vi "rad_Retrieve Image Wrapper.vi"(7 "Deployment Notifiers":T6, 8 "error in (no error)":errorcluster, 9 "AppImage Properties":T3, 10 "image file path":path, 11 "Target settings":T1={"Hostname"="", "Serial number"="", "Product name"="", "Product code"=0, "System status"="", "Credential type"=enum."None/Unlocked", "User added?"=FALSE, "Primary NIC"={"MAC address"="", "IP Address Request Mode"=2, "IP address"="", "Subnet mask"="", "Gateway"="", "DNS server"=""}} {"Primary NIC"."IP Address Request Mode" items=["Static"=1, "DHCP/Link-Local"=2, "Link-Local Only"=4, "DHCP Only"=8]}) -> (0 "error out":errorcluster, 3 "Canceled":bool)   [LabVIEW 2013]
uses:
  TypeDefs/rad_Deployment Progress Data Type.ctl
  TypeDefs/rad_Deployment Notifiers.ctl
  TypeDefs/rad_Deployment Status Data Type.ctl
  TypeDefs/rad_Application Image Properties.ctl
  TypeDefs/rad_FPGA Properties.ctl
  TypeDefs/rad_FPGA Flash Properties.ctl
  Targets/TypeDefs/rad_Target Information.ctl
  Targets/TypeDefs/rad_Target Network Settings.ctl
  <vilib>/nisyscfg/Software 1.2.ctl
  <vilib>/nisyscfg/Component Type.ctl
  <vilib>/nisyscfg/Create System Image (Folder).vi
  <vilib>/nisyscfg/Close (System).vi
  <vilib>/nisyscfg/nisyscfg.lvlib
panel:
  in  "Stop Checking for Events":bool
  out "Progress":T7 scale=0.0..100.0
  out "Status":string
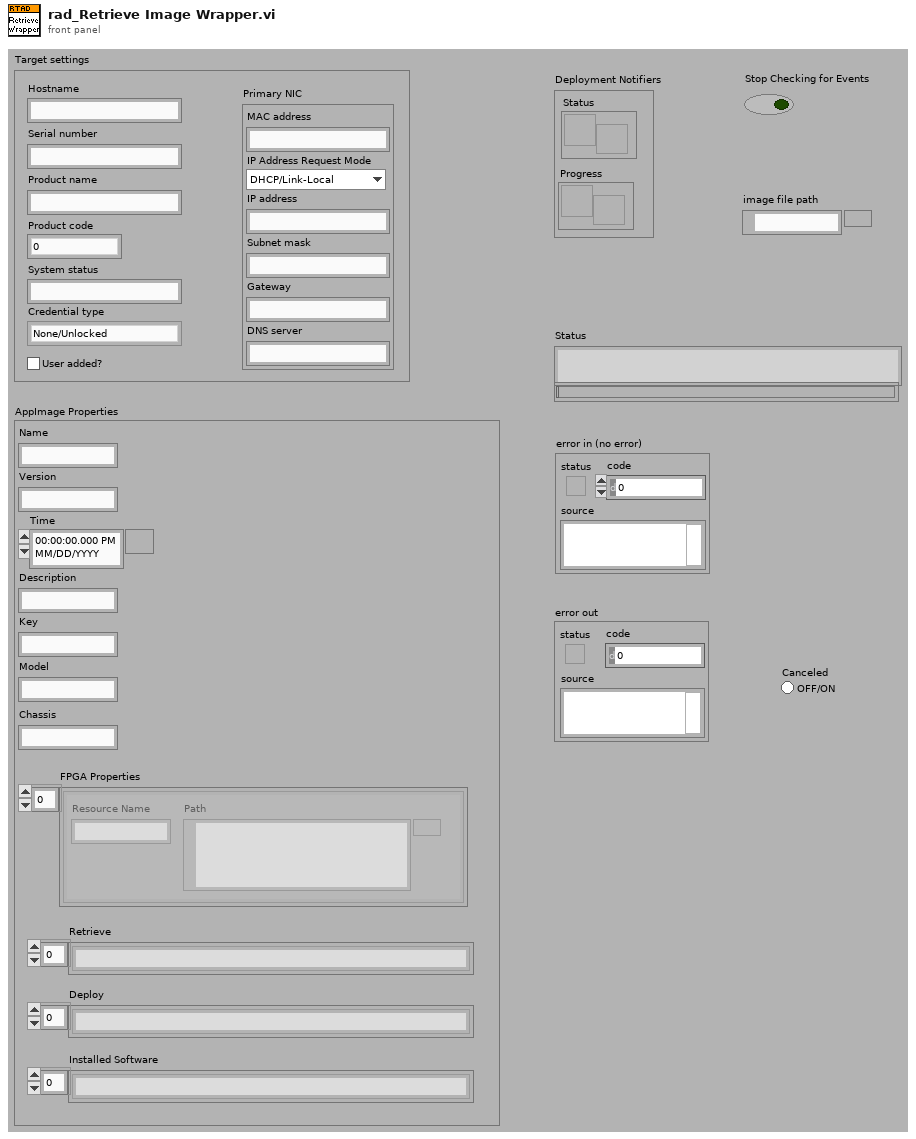
[diagram p1: front panel]
types:
  T1 = typedef "rad_Target Information.ctl" = cluster{"Hostname":string, "Serial number":string, "Product name":string, "Product code":i32, "System status":string, "Credential type":enum16{"None/Unlocked", "FTP Password", "NIAuth Credentials"}, "User added?":bool, "Primary NIC":T2}
  T2 = typedef "rad_Target Network Settings.ctl" = cluster{"MAC address":string, "IP Address Request Mode":i32, "IP address":string, "Subnet mask":string, "Gateway":string, "DNS server":string}
  T3 = typedef "rad_Application Image Properties.ctl" = cluster{"Name":string, "Version":string, "Time":timestamp, "Description":string, "Key":string, "Chassis":string, "FPGA Properties":T4, "Model":string, "Retrieve":string[], "Deploy":string[], "Installed Software":string[]}
  T4 = typedef "rad_FPGA Properties.ctl" = T5[]
  T5 = typedef "rad_FPGA Flash Properties.ctl" = cluster{"Resource Name":string, "Path":path}
  T6 = typedef "rad_Deployment Notifiers.ctl" = cluster{"Status":refnum<notifier>, "Progress":refnum<notifier>}
  T7 = typedef "rad_Deployment Progress Data Type.ctl" = i8
  T8 = typedef "nisyscfg.lvlib/Software 1.2.ctl" = cluster{"title":string, "description":string, "ID":string, "version":string, "component type":T9}
  T9 = typedef "nisyscfg.lvlib/Component Type.ctl" = u32
  T10 = enum32{"state changed", "beginning restart", "getting file", "putting file", "creating directory", "deleting file", "deleting directory", "enumerating file system", "renaming file", "current component", "operation progress", "downloading file", "unpacking file", "running install script"}
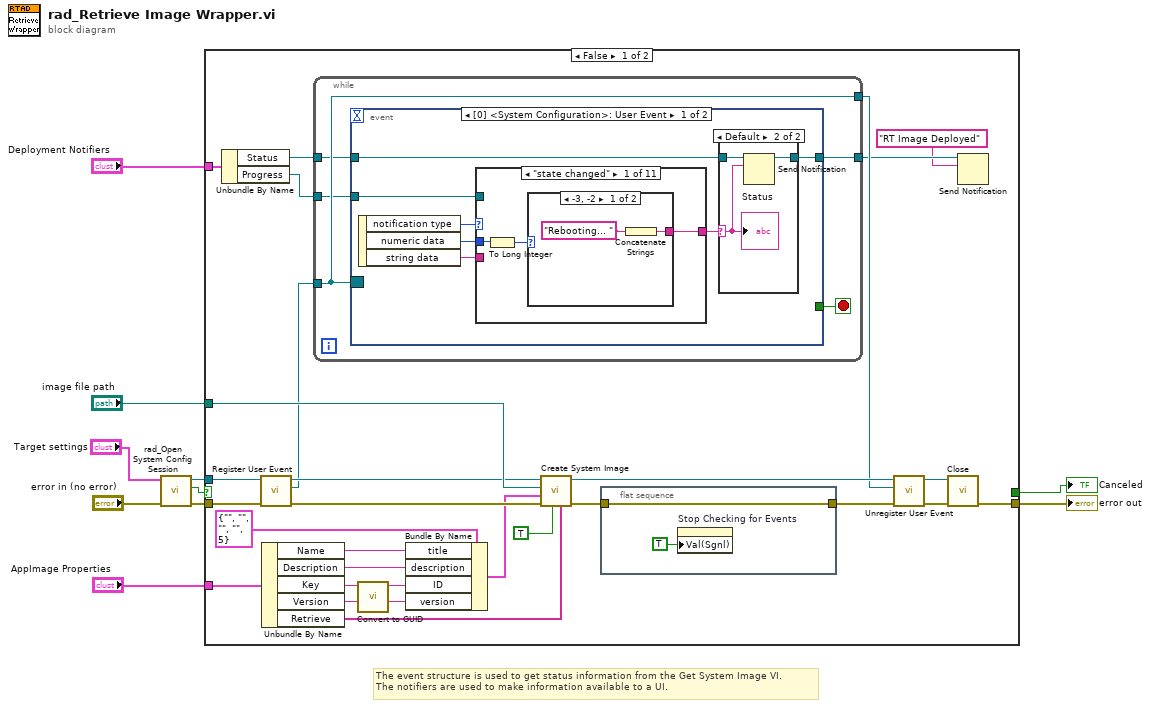
[diagram p0: block diagram]
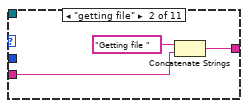
[diagram p4: hidden frame]
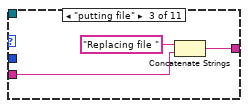
[diagram p5: hidden frame]
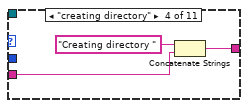
[diagram p6: hidden frame]
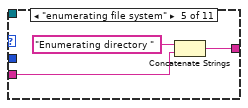
[diagram p7: hidden frame]
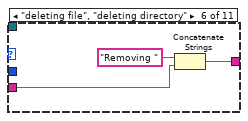
[diagram p8: hidden frame]
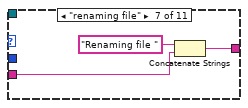
[diagram p9: hidden frame]
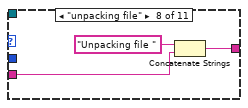
[diagram p10: hidden frame]
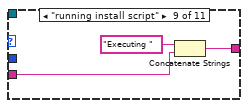
[diagram p11: hidden frame]
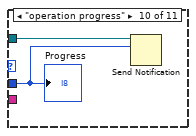
[diagram p12: hidden frame]
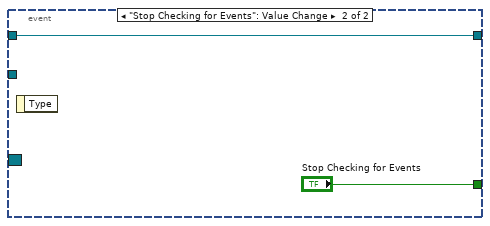
[diagram p14: hidden frame]
diagram:
  # "The event structure is used to get status information from the Get System Image VI. \nThe notifiers are used to make information available to a UI."
  n1 = call "rad_Open System Config Session.vi"("error in (no error)"="error in (no error)", "Target settings"="Target settings") -> ("error out"=w3:errorcluster, "Cancelled"=w2:bool, "Session out"=w4:refnum<k21>)  [unwired: 6 in, 1 out]
  n2 = case shown="False" w2 {
    selector: w2 -> [_ w90]
    tunnel: [w38 w91] -> w8
    tunnel: "image file path" -> [w37 _]
    tunnel: w4 -> [w36 _]
    tunnel: w3 -> [w35 w91]
    tunnel: "Deployment Notifiers" -> [w20 _]
    tunnel: "AppImage Properties" -> [w19 _]
    tunnel: [_ w90] -> w6
    frame False {
      n3 = Unbundle By Name(w20) -> ("Status"=w22:refnum<notifier>, "Progress"=w21:refnum<notifier>)
      n4 = call <vilib>:"Register User Event.vi"("error in (no error)"=w35, "Session in"=w36) -> ("error out"=w33:errorcluster, "Event Registration out"=w32:refnum<event-registration>, "Session out"=w34:refnum<k21>)  [unwired: 7 in]
      n5 = Unbundle By Name(w19) -> ("Name"=w16:string, "Description"=w15:string, "Key"=w12:string, "Version"=w14:string, "Retrieve"=w18:string[])
      n6 = while {
        tunnel: w32 -> [w45]
        tunnel: [w45] -> w28
        tunnel: w22 -> [w43]
        tunnel: [w42] -> w25
        tunnel: w21 -> [w41]
        stop <- w44 stop-if-true
        n7 = event shown="[0] <System Configuration>: User Event" {
          selector: w45 -> [_ _]
          dyn-events: _ -> [_ _]
          timeout: _ -> [_ _]
          tunnel: [_ "Stop Checking for Events"] -> w44
          tunnel: w43 -> [w48 w88]
          tunnel: [w47 w88] -> w42
          tunnel: w41 -> [w46 _]
          event User Event {
            n8 = event-data() -> ("notification type"=w52:T10, "numeric data"=w50:u32, "string data"=w51:string)  [unwired: 1 in]
            n9 = case shown="\"state changed\"" w52 {
              tunnel: [w57 w62 w65 w68 w71 w74 w77 w80 w83 _ _] -> w49
              tunnel: w51 -> [_ w63 w66 w69 w72 w75 w78 w81 w84 _ _]
              tunnel: w50 -> [w59 _ _ _ _ _ _ _ _ w86 _]
              tunnel: w46 -> [_ _ _ _ _ _ _ _ _ w87 _]
              frame "state changed" {
                n10 = To Long Integer(number=w59) -> (32bit integer=w58:i32)
                n11 = case shown="-3, -2" w58 {
                  tunnel: [w60 _] -> w57
                  frame -3, -2 {
                    n12 = Concatenate Strings("Rebooting... ") -> (w60:string)
                  }
                  frame Default {
                  }
                }
              }
              frame "getting file" {
                n13 = Concatenate Strings("Getting file " ("Status"), w63) -> (w62:string)
              }
              frame "putting file" {
                n14 = Concatenate Strings("Replacing file " ("Status"), w66) -> (w65:string)
              }
              frame "creating directory" {
                n15 = Concatenate Strings("Creating directory " ("Status"), w69) -> (w68:string)
              }
              frame "enumerating file system" {
                n16 = Concatenate Strings("Enumerating directory " ("Status"), w72) -> (w71:string)
              }
              frame "deleting file", "deleting directory" {
                n17 = Concatenate Strings("Removing " ("Status"), w75) -> (w74:string)
              }
              frame "renaming file" {
                n18 = Concatenate Strings("Renaming file " ("Status"), w78) -> (w77:string)
              }
              frame "unpacking file" {
                n19 = Concatenate Strings("Unpacking file " ("Status"), w81) -> (w80:string)
              }
              frame "running install script" {
                n20 = Concatenate Strings("Executing " ("Status"), w84) -> (w83:string)
              }
              frame "operation progress" {
                n21 = Send Notification(notification=w86, notifier=w87) -> ()  [unwired: 1 in, 2 out]
                "Progress" <- w86
              }
              frame Default {
              }
            }
            n22 = case shown="Default" w49 {
              selector: w49 -> [_ w55]
              tunnel: w48 -> [w53 w56]
              tunnel: [w53 w54] -> w47
              frame "" {
              }
              frame Default {
                n23 = Send Notification(notification=w55, notifier=w56) -> (notifier out=w54:refnum<notifier>)  [unwired: 1 in, 1 out]
                "Status" <- w55
              }
            }
          }
          event "Stop Checking for Events": Value Change {
            n24 = event-data() -> ()  [unwired: 1 in, 1 out]
          }
        }
      }
      n25 = call "Convert to GUID.vi"("Key"=w12) -> ("GUID"=w11:string)  [unwired: 10 in]
      n26 = Bundle By Name(cluster=T8 {"title"="", "description"="", "ID"="", "version"="", "component type"=5} ("image metadata"), "title"=w16, "description"=w15, "ID"=w11, "version"=w14) -> (w13:T8)
      n27 = call-poly <vilib>:"Create System Image.vi"("File and Directory Blacklist"=w18, "Overwrite (F)"=TRUE ("overwrite (F)"), "error in (no error)"=w33, "Image Metadata in"=w13, "Destination Folder"=w37, "Session in"=w34) -> ("error out"=w27:errorcluster, "Session out"=w29:refnum<k21>)  [unwired: 3 in, 1 out]
      n28 = flat-sequence {
        tunnel: w27 -> [w40]
        tunnel: [w40] -> w26
        frame #0 {
          n29 = property on="Stop Checking for Events" class="Bool (strict)"("Val(Sgnl)"=TRUE ("Stop Checking for Events")) -> ()  [unwired: 2 in, 2 out]
        }
      }
      n30 = call <vilib>:"Unregister User Event.vi"("error in (no error)"=w26, "Event Registration in"=w28, "Session in"=w29) -> ("error out"=w30:errorcluster, "Session out"=w31:refnum<k21>)  [unwired: 7 in]
      n31 = call-poly <vilib>:"Close.vi"("error in (no error)"=w30, "Session in"=w31) -> ("error out"=w38:errorcluster)  [unwired: 9 in]
      n32 = Send Notification(notification="RT Image Deployed", notifier=w25) -> ()  [unwired: 1 in, 2 out]
    }
    frame True {
    }
  }
  "error out" <- w8
  "Canceled" <- w6
